vi "102_Lip_Gap.vi"() -> ()   [LabVIEW 2015]
uses:
  <vilib>/vision/Measure.llb/Edge Options.ctl
  <vilib>/vision/Measure.llb/Edge Polarity.ctl
  <vilib>/vision/Image Controls.llb/IMAQ Image.ctl
  <vilib>/vision/NI_Vision_Development_Module.lvlib
panel:
  out "Final Point 2":cluster{"X":sgl, "Y":sgl}
  out "Final Point 1":cluster{"X":sgl, "Y":sgl}
  in  "Calibrated Image":T1
  in  "Angle from box":dbl
  in  "Measurement ROI 2":T2
  out "Real World Lip Gap 102":sgl
  out "error out":errorcluster
  in  "Process ROI 2":T3(ring)=enum."Get All Edges"
  in  "Edge Options ROI 2":T4={"Edge Polarity"=0, "Kernel Size"=3, "Width"=3, "Minimum Edge Strength"=10.0, "Interpolation Type"=enum."Bilinear Fixed", "Data Processing Method"=enum."Average"} {"Edge Polarity" items=["All Edges", "Rising Edges", "Falling Edges"]; "Minimum Edge Strength" format="%.2f"; "Width" step=2; "Kernel Size" step=2}
  in  "Scan Direction ROI 2":u16(ring) items=["Left To Right", "Right To Left", "Top To Bottom", "Bottom To Top"]
  in  "Step Size ROI 2":u32=5
  in  "Image In":T1(plugin-control)
  in  "error in (no error)":errorcluster
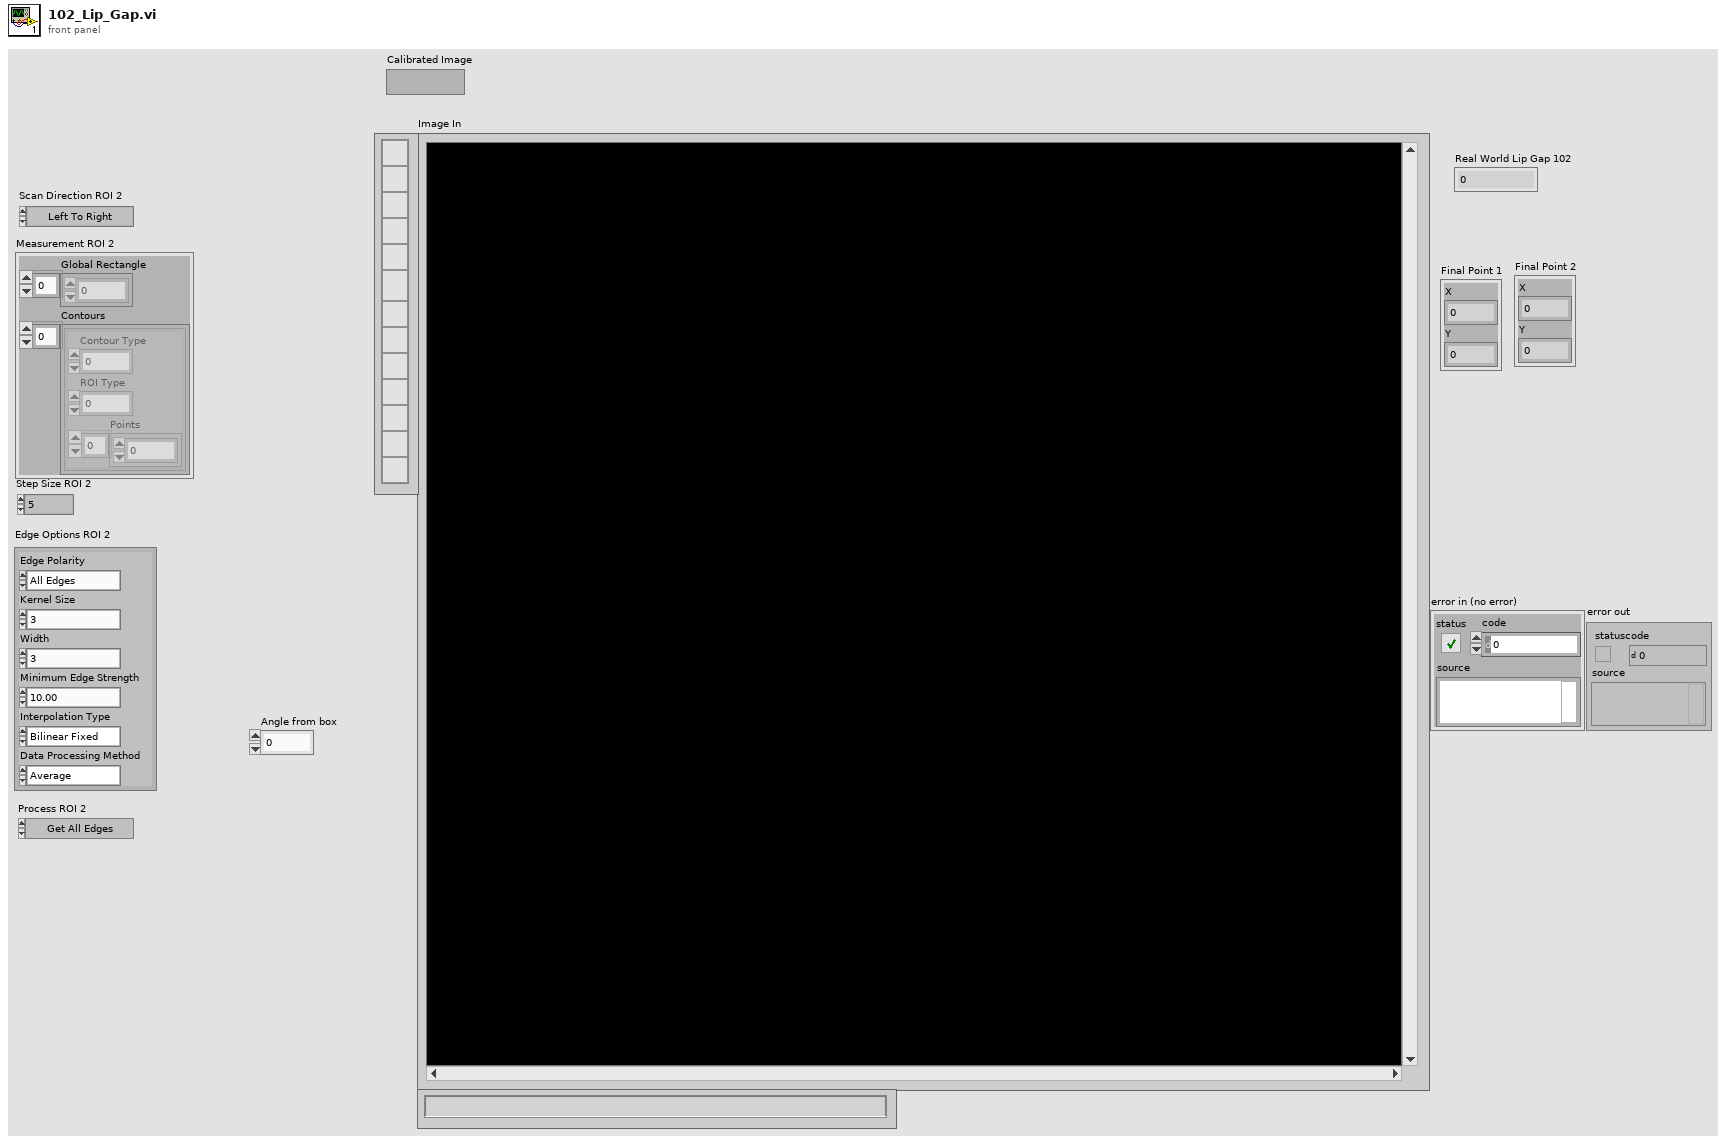
[diagram p1: front panel]
types:
  T1 = typedef "IMAQ Image.ctl" = refnum<image>
  T2 = cluster{"Global Rectangle":i32[], "Contours":cluster{"Contour Type":u32, "ROI Type":u32, "Points":i32[]}[]}
  T3 = enum16{"Get First Edge", "Get First + Last Edge", "Get All Edges", "Get Best Edge"}
  T4 = typedef "Edge Options.ctl" = cluster{"Edge Polarity":T5, "Kernel Size":u32, "Width":u32, "Minimum Edge Strength":sgl, "Interpolation Type":enum32{"Zero Order", "Bilinear", "Quadratic", "Cubic", "Bilinear Fixed"}, "Data Processing Method":enum32{"Average", "Median"}}
  T5 = typedef "Edge Polarity.ctl" = u32
  T6 = typedef "IMAQ Rectangle" = cluster{"Left":i32, "Top":i32, "Right":i32, "Bottom":i32, "Rotation":dbl}
  T7 = typedef "ROI Descriptor" = cluster{"Global Rectangle":i32[], "Contours":cluster{"ID":enum32{"External", "Internal"}, "Type":u32, "Coordinates":i32[]}[]}
  T8 = typedef "Search Line.ctl" = cluster{"Start Point":cluster{"X":sgl, "Y":sgl}, "End Point":cluster{"X":sgl, "Y":sgl}, "Edge Info":T9[], "Edge Map":dbl[], "Calibration Valid":bool}
  T9 = typedef "Edge New.ctl" = cluster{"Location (Pixel)":cluster{"X":sgl, "Y":sgl}, "Location (Real-World)":cluster{"X":sgl, "Y":sgl}, "Distance (Pixel)":dbl, "Distance (Real-World)":dbl, "Strength":dbl, "Noise":dbl, "Rising?":bool}
  T10 = typedef "IMAQ Line" = cluster{"Start X":i32, "Start Y":i32, "End X":i32, "End Y":i32}
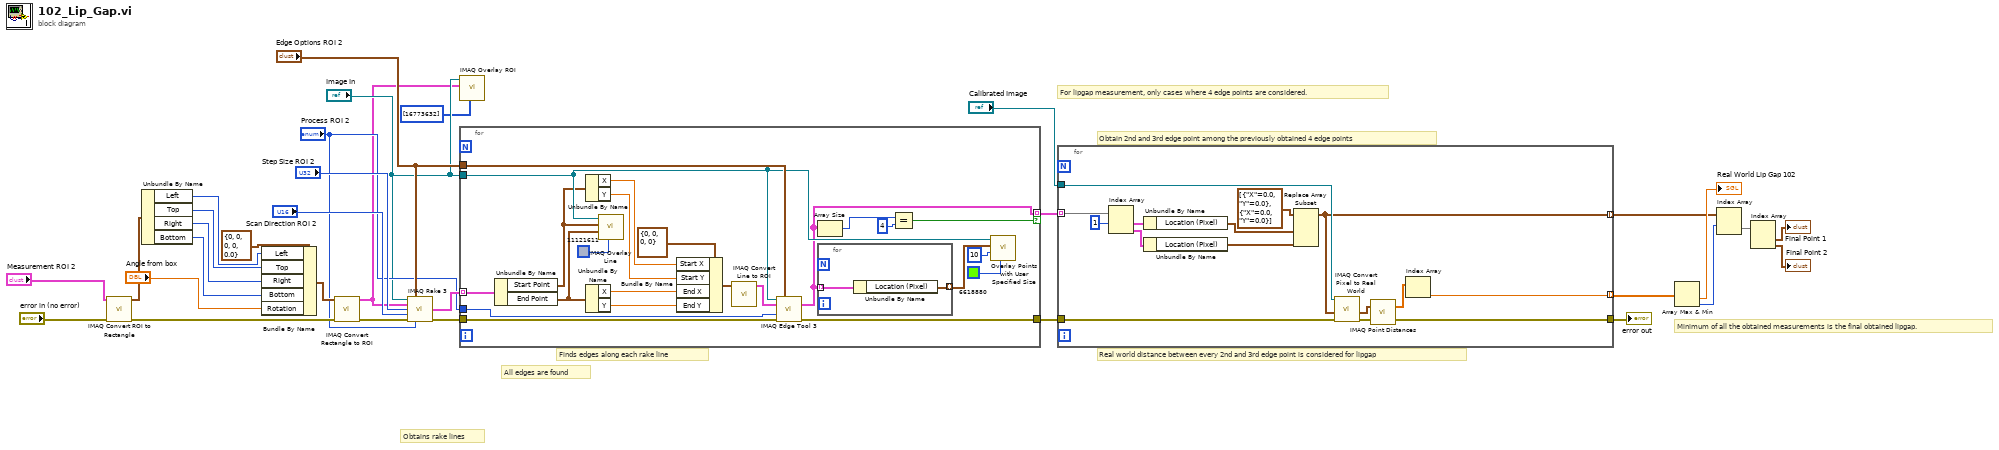
[diagram p0: block diagram]
diagram:
  # "Minimum of all the obtained measurements is the final obtained lipgap."
  # "Real world distance between every 2nd and 3rd edge point is considered for lipgap"
  # "Obtain 2nd and 3rd edge point among the previously obtained 4 edge points"
  # "For lipgap measurement, only cases where 4 edge points are considered."
  # "All edges are found"
  # "Finds edges along each rake line"
  # "Obtains rake lines"
  n1 = call "IMAQ Convert ROI to Rectangle"("error in (no error)"="error in (no error)", "ROI Descriptor"="Measurement ROI 2") -> ("error out"=w15:errorcluster, "Rectangle"=w25:T6)  [unwired: 7 in]
  n2 = Unbundle By Name(w25) -> ("Left"=w23:i32, "Top"=w22:i32, "Right"=w21:i32, "Bottom"=w20:i32)
  n3 = Bundle By Name(cluster=T6 {"Left"=0, "Top"=0, "Right"=0, "Bottom"=0, "Rotation"=0.0} ("Rectangle"), "Left"=w23, "Top"=w22, "Right"=w21, "Bottom"=w20, "Rotation"="Angle from box") -> (w18:T6)
  n4 = call "IMAQ Convert Rectangle to ROI"("error in (no error)"=w15, "Rectangle"=w18) -> ("error out"=w17:errorcluster, "ROI Descriptor"=w6:T7)  [unwired: 7 in]
  n5 = call "IMAQ Rake 3"("Image"="Image In", "Edge Options"="Edge Options ROI 2", "ROI Descriptor"=w6, "Step Size"="Step Size ROI 2", "Scan Direction"="Scan Direction ROI 2", "error in (no error)"=w17, "Process"="Process ROI 2") -> ("Search Lines"=w30:T8[], "error out"=w28:errorcluster)  [unwired: 5 in, 2 out]
  n6 = call "IMAQ Overlay ROI"("Colors (Green)"=u32[] [16773632], "ROI Descriptor"=w6, "Image"="Image In") -> ()  [unwired: 7 in, 2 out]
  n7 = for {
    tunnel: w30 -> [w55] mode=indexing
    tunnel: "Image In" -> [w42]
    tunnel: "Edge Options ROI 2" -> [w46]
    tunnel: w28 -> [w41]
    tunnel: [w40] -> w14
    tunnel: [w37] -> w27 mode=indexing if=w34
    tunnel: "Process ROI 2" -> [w33]
    n8 = Unbundle By Name(w55) -> ("Start Point"=w39:cluster{"X":sgl, "Y":sgl}, "End Point"=w38:cluster{"X":sgl, "Y":sgl})
    n9 = Unbundle By Name(w39) -> ("X"=w52:sgl, "Y"=w51:sgl)
    n10 = Unbundle By Name(w38) -> ("X"=w50:sgl, "Y"=w49:sgl)
    n11 = call "IMAQ Overlay Line"("Color"=u32 11121611, "End Point"=w38, "Start Point"=w39, "Image"=w42) -> ()  [unwired: 6 in, 2 out]
    n12 = Bundle By Name(cluster=T10 {"Start X"=0, "Start Y"=0, "End X"=0, "End Y"=0} ("Line"), "Start X"=w52, "Start Y"=w51, "End X"=w50, "End Y"=w49) -> (w48:T10)
    n13 = call "IMAQ Convert Line to ROI"("Line"=w48) -> ("ROI Descriptor"=w47:T7)  [unwired: 8 in, 1 out]
    n14 = call "IMAQ Edge Tool 3"("Image"=w42, "Edge Options"=w46, "ROI Descriptor"=w47, "Process"=w33, "error in (no error)"=w41) -> ("Edge Information"=w37:T9[], "error out"=w40:errorcluster)  [unwired: 6 in, 3 out]
    n15 = Array Size(array=w37) -> (size(s)=w36:i32)
    n16 = for {
      tunnel: w37 -> [w57] mode=indexing
      tunnel: [w56] -> w43 mode=indexing
      n17 = Unbundle By Name(w57) -> ("Location (Pixel)"=w56:cluster{"X":sgl, "Y":sgl})
    }
    n18 = Equal?(x=w36, y=4) -> (x = y?=w34:bool)
    n19 = call "Overlay Points with User Specified Size.vi"("Color"=u32 6618880, "Point Diameter (5)"=u32 10, "Points"=w43, "Image In"=w42) -> ()  [unwired: 6 in, 2 out]
  }
  n20 = for {
    tunnel: w27 -> [w59] mode=indexing
    tunnel: w14 -> [w65]
    tunnel: "Calibrated Image" -> [w63]
    tunnel: [w61] -> w12 mode=indexing
    tunnel: [w60] -> w11
    tunnel: [w58] -> w5 mode=indexing
    n21 = Index Array(array=w59, index #1=1 ("index")) -> (element #1=w71:T9, element #2=w70:T9)  [unwired: 1 in]
    n22 = Unbundle By Name(w71) -> ("Location (Pixel)"=w68:cluster{"X":sgl, "Y":sgl})
    n23 = Unbundle By Name(w70) -> ("Location (Pixel)"=w67:cluster{"X":sgl, "Y":sgl})
    n24 = Replace Array Subset(array=cluster{"X":sgl, "Y":sgl}[] [{"X"=0.0, "Y"=0.0}, {"X"=0.0, "Y"=0.0}], new element #1=w68, new element #2=w67) -> (w58:cluster{"X":sgl, "Y":sgl}[])  [unwired: 2 in]
    n25 = call "IMAQ Convert Pixel to Real World"("error in (no error)"=w65, "Array of Pixel Coordinates"=w58, "Calibrated Image"=w63) -> ("error out"=w64:errorcluster, "Array of Real World Coordinates"=w66:cluster{"X":sgl, "Y":sgl}[])  [unwired: 3 in, 4 out]
    n26 = call "IMAQ Point Distances"("Points"=w66, "error in (no error)"=w64) -> ("Distances"=w62:sgl[], "error out"=w60:errorcluster)  [unwired: 3 in]
    n27 = Index Array(array=w62) -> (element=w61:sgl)  [unwired: 1 in]
  }
  "error out" <- w11
  n28 = Array Max & Min(array=w12) -> (min value=→"Real World Lip Gap 102":sgl, min index (indices)=w4:i32)  [unwired: 2 out]
  n29 = Index Array(array=w5, index (row)=w4) -> (element=w3:cluster{"X":sgl, "Y":sgl}[])  [unwired: 1 in]
  n30 = Index Array(array=w3) -> (element #1=→"Final Point 1":cluster{"X":sgl, "Y":sgl}, element #2=→"Final Point 2":cluster{"X":sgl, "Y":sgl})  [unwired: 2 in]
